vi "Buzz Alert.vi"(7 "Buzz":bool, 8 "error out":errorcluster, 9 "limitation value":dbl, 10 "input value":dbl, 11 "VISA resource 2":refnum<visa-resource-name>) -> (0 "error out 2":errorcluster, 3 "VISA resource 3":refnum<visa-resource-name>)   [LabVIEW 2011]
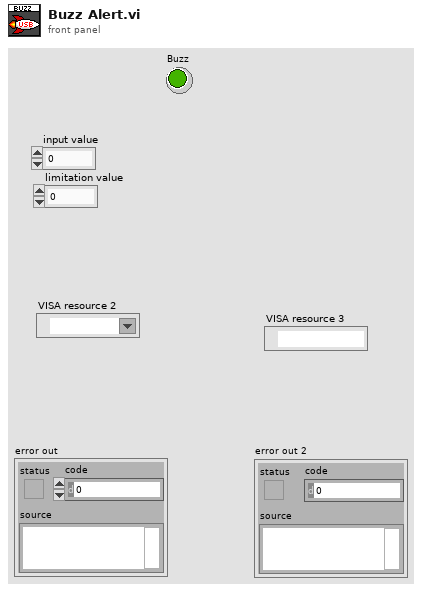
[diagram p1: front panel]
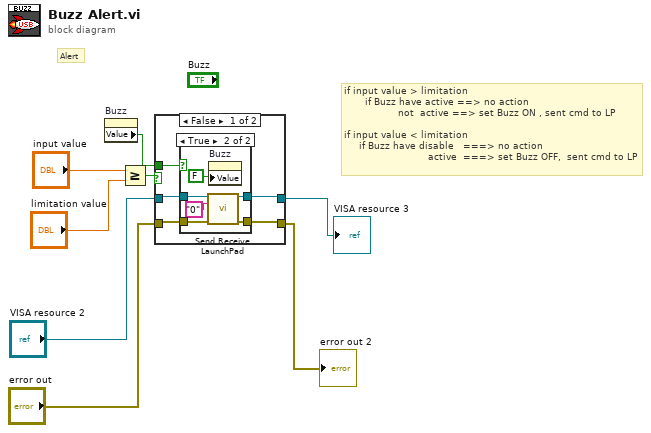
[diagram p0: block diagram]
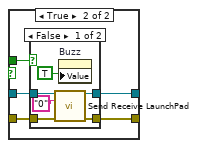
[diagram p3: hidden frame]
diagram:
  # "if input value > limitation \n       if Buzz have active ==> no action \n                  not  active ==> set Buzz ON , sent cmd to LP \n\nif input value < limitation\n     if Buzz have disable   ===> no action\n                            active  ===> set Buzz OFF,  sent cmd to LP"
  # "Alert"
  n1 = property on="Buzz" class="Bool (strict)"() -> ("Value"=w7:bool)  [unwired: 2 in, 2 out]
  n2 = Greater Or Equal?(x="input value", y="limitation value") -> (x >= y?=w8:bool)
  n3 = case shown="False" w8 {
    tunnel: "VISA resource 2" -> [w12 w26]
    tunnel: [w10 w25] -> w2
    tunnel: "error out" -> [w11 w24]
    tunnel: [w9 w23] -> w1
    tunnel: w7 -> [w13 w22]
    frame False {
      n4 = case shown="True" w13 {
        tunnel: w12 -> [w15 w19]
        tunnel: w11 -> [w14 w18]
        tunnel: [w15 w17] -> w10
        tunnel: [w14 w16] -> w9
        frame False {
        }
        frame True {
          n5 = call "Send Receive LaunchPad.vi"("VISA resource"=w19, "write buffer"="0", "error in"=w18) -> ("VISA resource 2"=w17:refnum<visa-resource-name>, "error out"=w16:errorcluster)  [unwired: 10 in, 1 out]
          n6 = property on="Buzz" class="Bool (strict)"("Value"=FALSE) -> ()  [unwired: 2 in, 2 out]
        }
      }
    }
    frame True {
      n7 = case shown="False" w22 {
        tunnel: w26 -> [w31 w34]
        tunnel: [w28 w34] -> w25
        tunnel: w24 -> [w30 w33]
        tunnel: [w29 w33] -> w23
        frame False {
          n8 = call "Send Receive LaunchPad.vi"("VISA resource"=w31, "write buffer"="0", "error in"=w30) -> ("VISA resource 2"=w28:refnum<visa-resource-name>, "error out"=w29:errorcluster)  [unwired: 10 in, 1 out]
          n9 = property on="Buzz" class="Bool (strict)"("Value"=TRUE) -> ()  [unwired: 2 in, 2 out]
        }
        frame True {
        }
      }
    }
  }
  "VISA resource 3" <- w2
  "error out 2" <- w1
